vi "Save to LVTest File.vi"(8 "error in (no error)":errorcluster, 10 "LVTest File Path":path, 11 "LUnit Test Vector In":refnum<class "LUnit Test Vector.lvclass">) -> (0 "error out":errorcluster, 3 "LUnit Test Vector Out":refnum<class "LUnit Test Vector.lvclass">)   [LabVIEW 2020, in "LUnit Test Vector.lvclass"]
doc: "Saves the current test vector to a file formated using the LVTest file format."
uses:
  LUnit Test Vector.lvclass
  LUnit Test Vector.lvclass/LUnit Test Vector.ctl
  Private/SubVIs/Variant with Type Information to Strings.vi
  <vilib>/Utility/libraryn.llb/Get File Extension.vi
  <vilib>/Utility/Data Type/Get Type Information.vi
  <vilib>/Utility/error.llb/Error Cluster From Error Code.vi
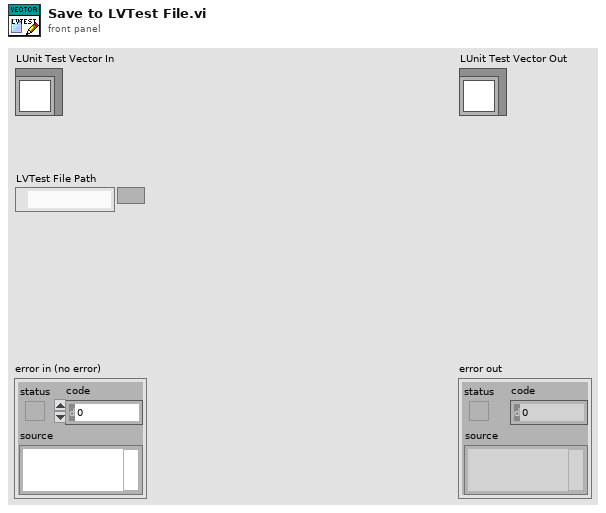
[diagram p1: front panel]
types:
  T1 = enum16{"open", "replace", "create", "open or create", "replace or create", "replace or create with confirmation"}
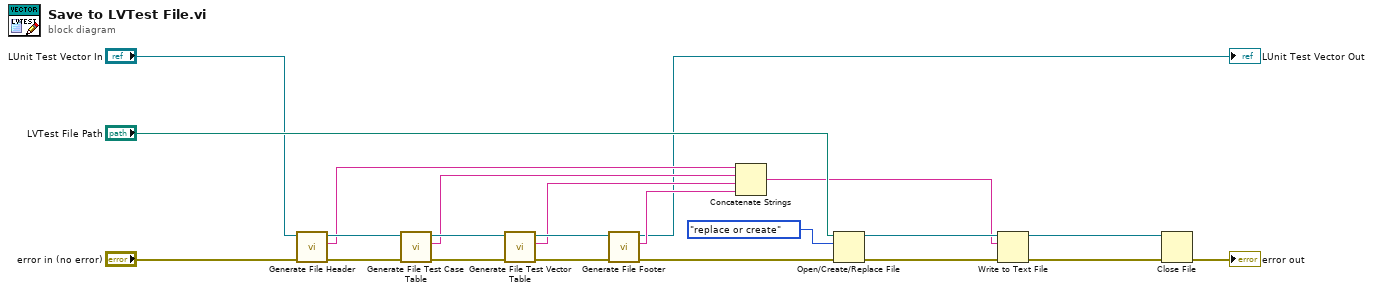
[diagram p0: block diagram]
diagram:
  n1 = call "Generate File Header.vi"("error in (no error)"="error in (no error)", "LUnit Test Vector in"="LUnit Test Vector In") -> ("error out"=w20:errorcluster, "Header"=w15:string, "LUnit Test Vector out"=w21:refnum<class "LUnit Test Vector.lvclass">)  [unwired: 7 in]
  n2 = call "Generate File Test Case Table.vi"("error in (no error)"=w20, "LUnit Test Vector in"=w21) -> ("error out"=w18:errorcluster, "Test Case Table"=w14:string, "LUnit Test Vector out"=w19:refnum<class "LUnit Test Vector.lvclass">)  [unwired: 7 in]
  n3 = call "Generate File Test Vector Table.vi"("error in (no error)"=w18, "LUnit Test Vector in"=w19) -> ("error out"=w16:errorcluster, "Test Vector Table"=w13:string, "LUnit Test Vector out"=w17:refnum<class "LUnit Test Vector.lvclass">)  [unwired: 7 in]
  n4 = call "Generate File Footer.vi"("error in (no error)"=w16, "LUnit Test Vector in"=w17) -> ("error out"=w7:errorcluster, "Header"=w12:string, "LUnit Test Vector out"=→"LUnit Test Vector Out":refnum<class "LUnit Test Vector.lvclass">)  [unwired: 7 in]
  n5 = Concatenate Strings(w15, w14, w13, w12) -> (w5:string)
  n6 = Open/Create/Replace File(file path (use dialog)="LVTest File Path", error in=w7, operation (0:open)=T1."replace or create") -> (refnum out=w11:refnum<file>, error out=w10:errorcluster)  [unwired: 3 in, 1 out]
  n7 = Write to Text File(file (use dialog)=w11, text=w5, error in=w10) -> (refnum out=w9:refnum<file>, error out=w8:errorcluster)  [unwired: 1 in, 1 out]
  n8 = Close File(refnum=w9, error in=w8) -> (error out=→"error out":errorcluster)  [unwired: 1 out]
